vi "Create Buffer.vi"(7 "Buffer Size (10k)":i32=10000 format="%.0p", 8 "error in (no error)":errorcluster) -> (0 "error out":errorcluster)   [LabVIEW 2025, in "Automotive Ethernet Bus Monitor UI.lvlib"]
doc: "Create the Table Buffer."
uses:
  Automotive Ethernet Bus Monitor UI.lvlib
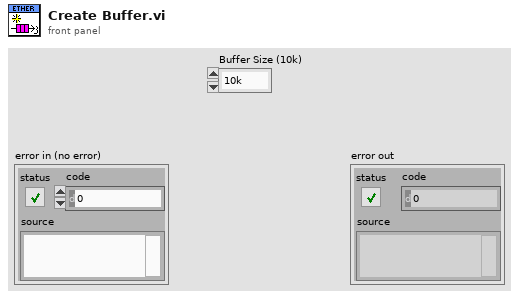
[diagram p1: front panel]
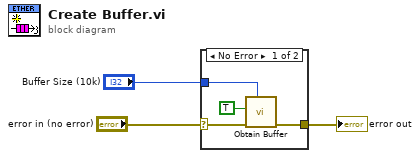
[diagram p0: block diagram]
diagram:
  n1 = case shown="No Error" "error in (no error)" {
    selector: "error in (no error)" -> [w6 w8]
    tunnel: [w7 w8] -> w2
    tunnel: "Buffer Size (10k)" -> [w4 _]
    frame No Error {
      n2 = call "Obtain Buffer.vi"("Buffer Size (10k)"=w4, "error in (no error)"=w6, "Create (F)"=TRUE ("create if not found? (T)")) -> ("error out"=w7:errorcluster)  [unwired: 7 in, 1 out]
    }
    frame Error {
    }
  }
  "error out" <- w2
